vi "TrimString.vi"(8 "string 4":string, 9 "string 3":string, 10 "string 2":string, 11 "string":string) -> (0 "trimmed string 4":string, 1 "trimmed string 3":string, 2 "trimmed string 2":string, 3 "trimmed string":string)   [LabVIEW 2012]
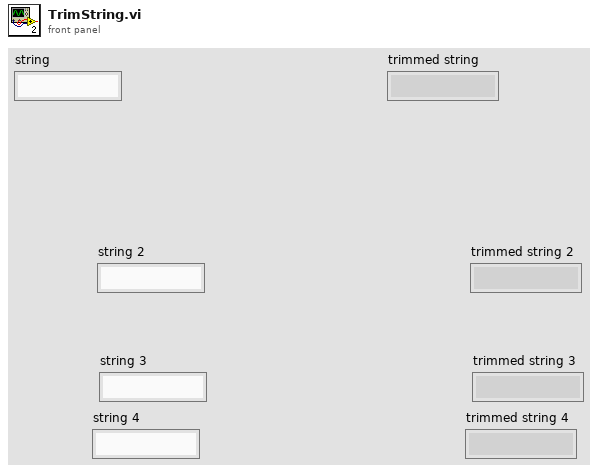
[diagram p1: front panel]
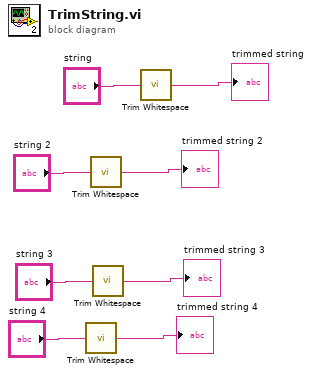
[diagram p0: block diagram]
diagram:
  n1 = call <vilib>:"Trim Whitespace.vi"("string"="string 4") -> ("trimmed string"=→"trimmed string 4":string)  [unwired: 1 in]
  n2 = call <vilib>:"Trim Whitespace.vi"("string"="string 2") -> ("trimmed string"=→"trimmed string 2":string)  [unwired: 1 in]
  n3 = call <vilib>:"Trim Whitespace.vi"("string"="string 3") -> ("trimmed string"=→"trimmed string 3":string)  [unwired: 1 in]
  n4 = call <vilib>:"Trim Whitespace.vi"("string"="string") -> ("trimmed string"=→"trimmed string":string)  [unwired: 1 in]
